vi "IPC.vi"(1 "Coerced Values":cluster{"Max":dbl, "Min":dbl, "Coerce?":bool}, 2 "Stop Changing":bool, 3 "Initilization":dbl, 4 "Reset":bool, 5 "Multiplier":dbl=1.0, 6 "Value":dbl) -> (0 "IPCed":dbl)   [LabVIEW 2019]
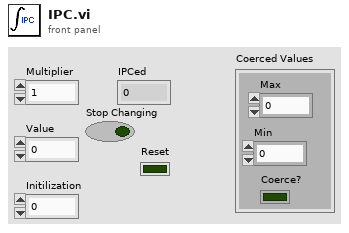
[diagram p1: front panel]
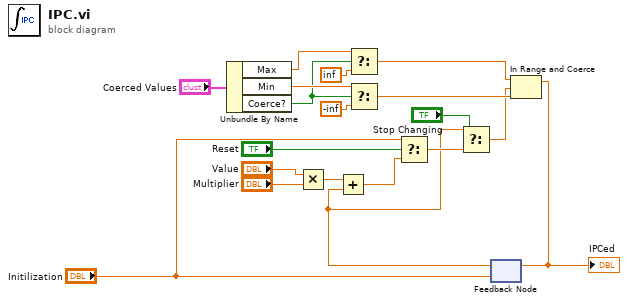
[diagram p0: block diagram]
diagram:
  n1 = Unbundle By Name("Coerced Values") -> ("Max"=w15:dbl, "Min"=w14:dbl, "Coerce?"=w13:bool)
  n2 = Multiply(x="Value", y="Multiplier") -> (x*y=w19:dbl)
  n3 = Select(t=w15, s=w13, f=inf) -> (s? t:f=w10:dbl)
  n4 = Select(t=w14, s=w13, f=-inf) -> (s? t:f=w9:dbl)
  n5 = feedback #1("Initilization") -> (w2:dbl)
  n6 = Add(x=w19, y=w2) -> (x+y=w6:dbl)
  n7 = Select(t="Initilization", s="Reset", f=w6) -> (s? t:f=w4:dbl)
  n8 = Select(t=w2, s="Stop Changing", f=w4) -> (s? t:f=w3:dbl)
  n9 = In Range and Coerce(upper limit=w10, x=w3, lower limit=w9) -> (coerced(x)=w8:dbl)  [unwired: 1 out]
  "IPCed" <- w8
  n10 = feedback-in #1(w8) -> ()
